vi "get rid of extra on motor.vi"(1 "Numeric":dbl) -> (0 "extra":dbl)   [LabVIEW 2013]
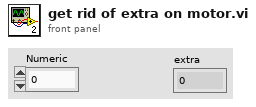
[diagram p1: front panel]
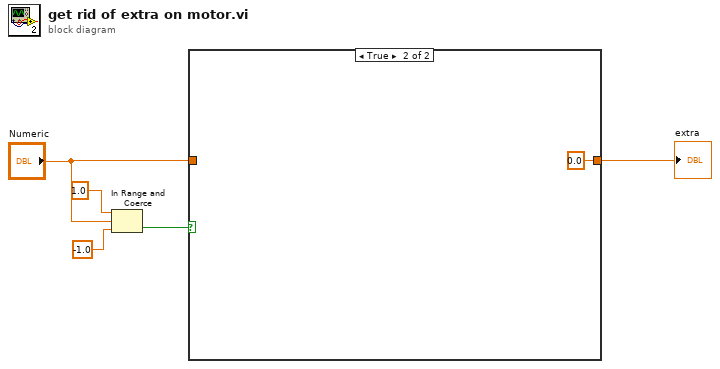
[diagram p0: block diagram]
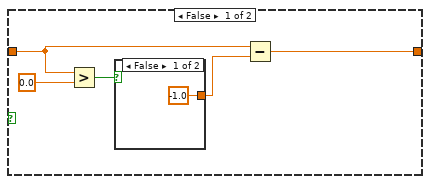
[diagram p2: hidden frame]
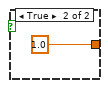
[diagram p3: hidden frame]
diagram:
  n1 = In Range and Coerce(upper limit=1.0, x="Numeric", lower limit=-1.0) -> (In Range?=w1:bool)  [unwired: 1 out]
  n2 = case shown="True" w1 {
    tunnel: [w6 0.0] -> w5
    tunnel: "Numeric" -> [w8 _]
    frame False {
      n3 = Greater?(x=w8, y=0.0) -> (0:w9:bool)
      n4 = case shown="False" w9 {
        tunnel: [-1.0 ("y") 1.0 ("y")] -> w7
        frame False {
        }
        frame True {
        }
      }
      n5 = Subtract(x=w8, y=w7) -> (x-y=w6:dbl)
    }
    frame True {
    }
  }
  "extra" <- w5
